vi "Różnica azymutów sprowadzona do zakresu +-180 stopni.vi"(9 "Azymut robota":dbl(slide) scale=0.0..360.0, 10 "Azymut - zadany":dbl(slide) scale=0.0..360.0) -> (2 "az_z - az_r":dbl)   [LabVIEW 2012, in "Biblioteka moduł map v3.lvlib" / "Matematyczne.lvlib"]
uses:
  Matematyczne.lvlib
panel:
  # "<-180,180>"
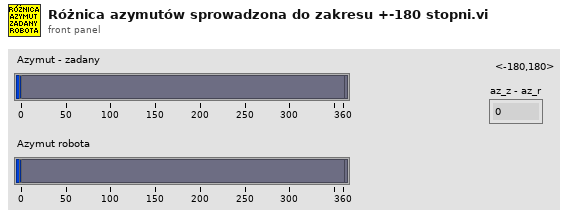
[diagram p1: front panel]
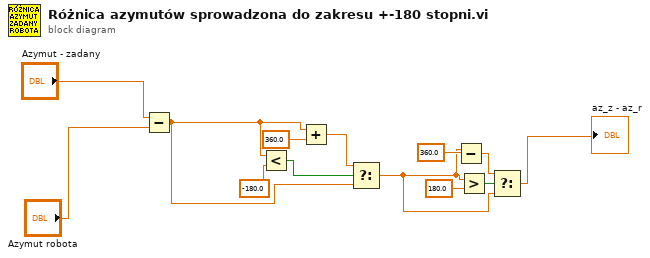
[diagram p0: block diagram]
diagram:
  n1 = Subtract(x="Azymut - zadany", y="Azymut robota") -> (x-y=w7:dbl)
  n2 = Less?(x=w7, y=-180.0) -> (x < y?=w12:bool)
  n3 = Add(x=w7, y=360.0) -> (x+y=w10:dbl)
  n4 = Select(t=w10, s=w12, f=w7) -> (s? t:f=w4:dbl)
  n5 = Subtract(x=w4, y=360.0) -> (x-y=w5:dbl)
  n6 = Greater?(x=w4, y=180.0) -> (0:w8:bool)
  n7 = Select(t=w5, s=w8, f=w4) -> (s? t:f=→"az_z - az_r":dbl)
